vi "dfd_nMAC_DelayNwReset.vi"(1 "reset":bool, 2 "data in":bool) -> (7 "data out":bool)   [LabVIEW 2017]
doc: "Number of delay must be less than 64."
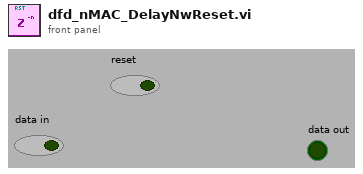
[diagram p1: front panel]
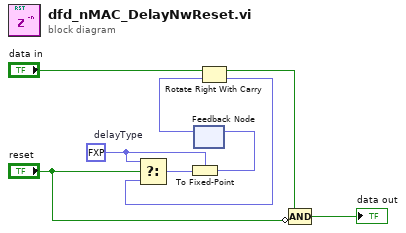
[diagram p0: block diagram]
diagram:
  w1 = fxp<+,1,1> 0.0  # delayType
  n1 = feedback #1() -> (w5:fxp<+,1,1>)  [unwired: 1 out]
  n2 = Rotate Right With Carry(2:w5, 3:"data in") -> (0:w4:fxp<+,1,1>, 1:w8:bool)
  n3 = Select(t=w1, s="reset", f=w4) -> (s? t:f=w3:fxp<+,1,1>)
  n4 = To Fixed-Point(fixed-point type=w1, number=w3) -> (fixed-point=w2:fxp<+,1,1>)
  n5 = feedback-in #1(w2) -> ()
  n6 = Compound Arithmetic op=AND(w8, invert "reset") -> (→"data out":bool)
